vi "Send Python to LabVIEW message.vi"(7 "Server Alias":string, 8 "error in (no error)":errorcluster, 11 "Message":T1={"Command"="zxcvbnm,", "Data"=["asdfghjk", "qwertyui"], "Script ID"=0, "LabVIEW Server ID"="zxcvbnm,", "Python Message ID"=0}) -> (0 "error out":errorcluster)   [LabVIEW 2013, in "TS.lvlib"]
doc: "We use the callback VI dynamically, to keep the TS.lvlib separate from the user's framework.\nWe send a message received from Python to the LV side."
uses:
  TS.lvlib
  LabVIEW Python Connector Message.ctl
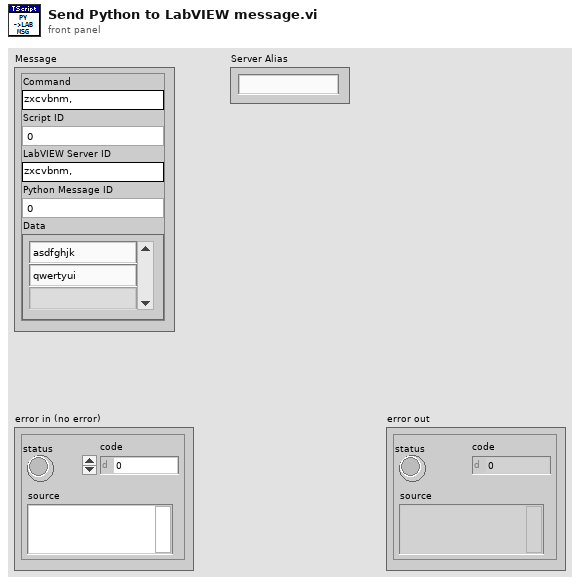
[diagram p1: front panel]
types:
  T1 = typedef "TS.lvlib/LabVIEW Python Connector Message.ctl" = cluster{"Command":string, "Data":string[], "Script ID":i64, "LabVIEW Server ID":string, "Python Message ID":i32}
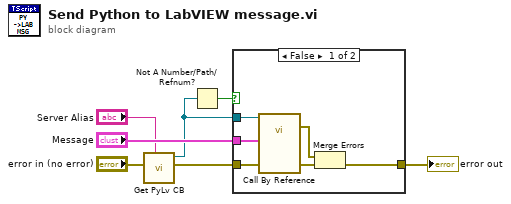
[diagram p0: block diagram]
diagram:
  n1 = call "Get PyLv CB.vi"("Server Alias"="Server Alias", "Error In"="error in (no error)") -> ("Error Out"=w3:errorcluster, "VI Refnum"=w2:refnum<vi>)  [unwired: 8 in]
  n2 = Not A Number/Path/Refnum?(number/path/refnum=w2) -> (NaN/Path/Refnum?=w6:bool)
  n3 = case shown="False" w6 {
    tunnel: w3 -> [w10 w14]
    tunnel: [w13 w14] -> w7
    tunnel: "Message" -> [w11 _]
    tunnel: w2 -> [w12 _]
    frame False {
      n4 = call-by-ref "?"(reference=w12, "error in (no error)"=w10, "Message to LabVIEW App"=w11) -> (error out=w8:errorcluster, 0:"error out"=w9:errorcluster)  [unwired: 10 in, 1 out]
      n5 = Merge Errors(w8, w9) -> (w13:errorcluster)
    }
    frame True {
      # "Not a valid reference\nNo op"
    }
  }
  "error out" <- w7
